vi "Logowanie_subvi.vi"() -> ()   [LabVIEW 2012]
panel:
  out "error out":errorcluster
  in  "error in (no error)":errorcluster
  out "login:out":string
  out "hasło:out":string
  in  "Wpisz login:":string
  in  "Wpisz hasło:":string
  in  "continue":bool
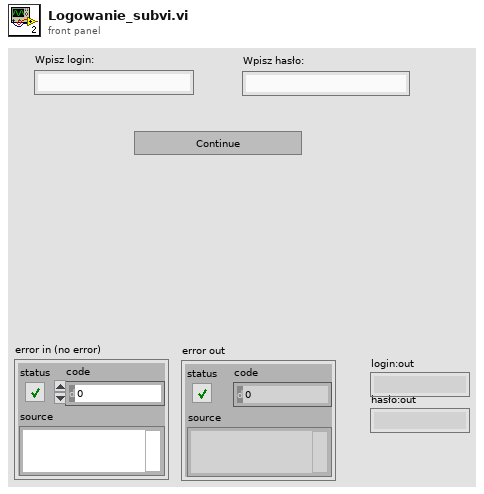
[diagram p1: front panel]
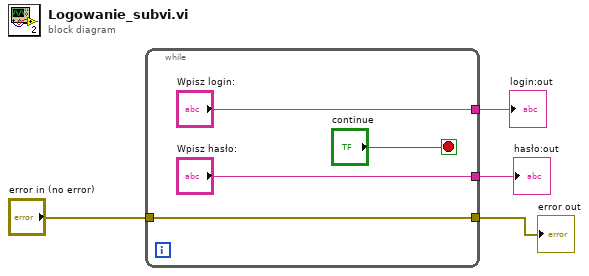
[diagram p0: block diagram]
diagram:
  n1 = while {
    tunnel: ["Wpisz login:"] -> w3
    tunnel: ["Wpisz hasło:"] -> w4
    tunnel: [w5] -> w2
    tunnel: "error in (no error)" -> [w5]
    stop <- "continue" stop-if-true
  }
  "hasło:out" <- w4
  "login:out" <- w3
  "error out" <- w2
